vi "Execute.vi"(8 "error in (no error)":errorcluster, 11 "Node in":refnum<class "bt_Failure.lvclass">) -> (0 "error out":errorcluster, 1 "Status":T1, 3 "Node out":refnum<class "bt_Failure.lvclass">)   [LabVIEW 2021, in "BT.lvlib" / "bt_Failure.lvclass"]
uses:
  bt_Failure.lvclass
  bt_Failure.lvclass/bt_Failure.ctl
  abs_Node/Status.ctl
  abs_Node/bt_Node.lvclass
  Support/Decorator/bt_Decorator.lvclass
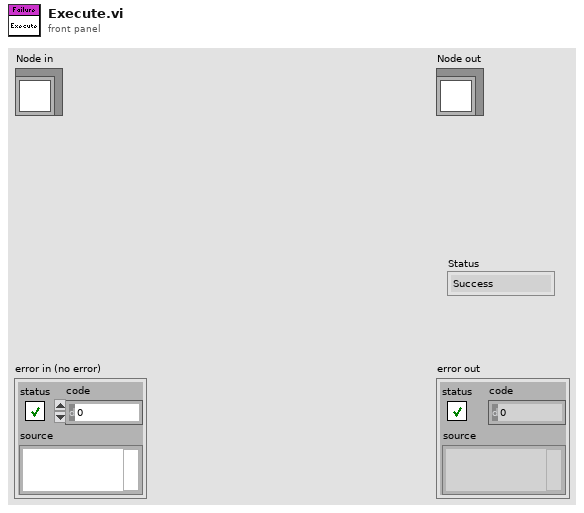
[diagram p1: front panel]
types:
  T1 = typedef "BT.lvlib/bt_Node.lvclass/Status.ctl" = enum16{"Success", "Failure", "Running"}
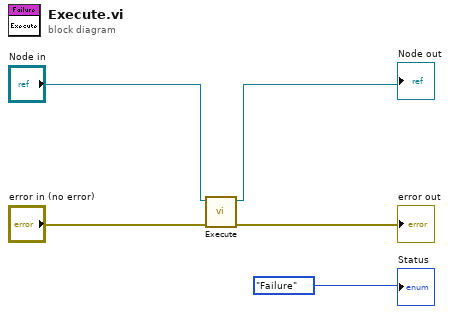
[diagram p0: block diagram]
diagram:
  n1 = call-parent "Execute.vi"("error in (no error)"="error in (no error)", "Node in"="Node in") -> ("error out"=→"error out":errorcluster, "Node out"=→"Node out":refnum<class "bt_Failure.lvclass">)  [unwired: 7 in, 1 out]
  "Status" <- Status."Failure" ("Status")
